vi "ble_check_payload_error.vi"(8 "error in (no error)":errorcluster, 10 "error source":string, 11 "payload":u8[](array[numeric])) -> (0 "error out":errorcluster, 3 "success?":bool)   [LabVIEW 2015]
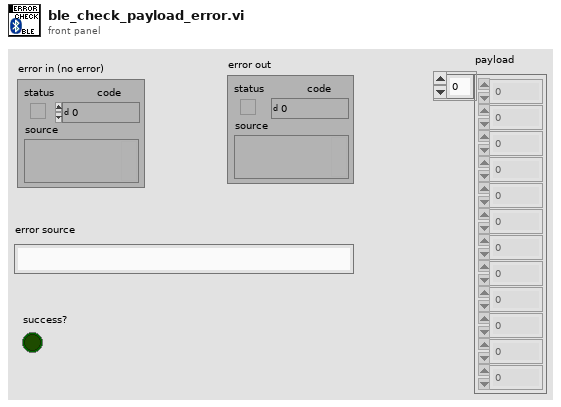
[diagram p1: front panel]
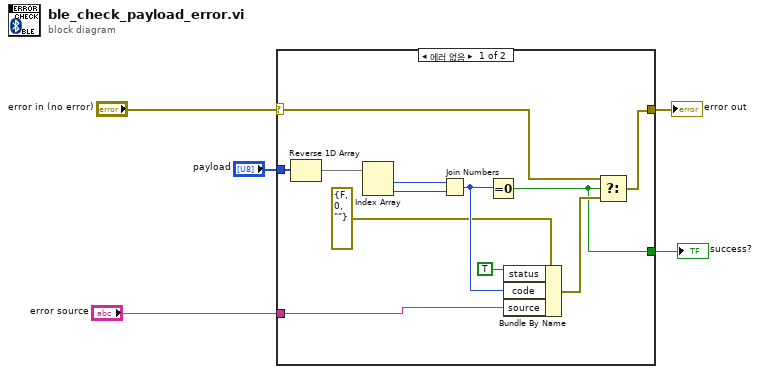
[diagram p0: block diagram]
diagram:
  n1 = case shown="에러 없음" "error in (no error)" {
    selector: "error in (no error)" -> [w12 w18]
    tunnel: "payload" -> [w17 _]
    tunnel: [w13 w18] -> w4
    tunnel: "error source" -> [w9 _]
    tunnel: [w6 _] -> w1
    frame No Error {
      n2 = Reverse 1D Array(array=w17) -> (reversed array=w16:u8[])
      n3 = Index Array(array=w16) -> (element #1=w14:u8, element #2=w15:u8)  [unwired: 2 in]
      n4 = Join Numbers(hi=w14, lo=w15) -> ((hi.lo)=w10:u16)
      n5 = Equal To 0?(x=w10) -> (x = 0?=w6:bool)
      n6 = Bundle By Name(cluster=errorcluster {"status"=FALSE, "code"=0, "source"=""} ("error in (no error)"), "status"=TRUE, "code"=w10, "source"=w9) -> (w7:errorcluster)
      n7 = Select(t=w12, s=w6, f=w7) -> (s? t:f=w13:errorcluster)
    }
    frame Error {
    }
  }
  "error out" <- w4
  "success?" <- w1
